vi "process.vi"(8 "error in (no error)":errorcluster, 9 "Calling VI Reference i":refnum<vi>, 10 "GObj Refnum":refnum<vi>, 11 "Loop in":refnum<class "Loop.lvclass">) -> (0 "error out":errorcluster, 3 "Loop out":refnum<class "Loop.lvclass">)   [LabVIEW 2016, in "Loop.lvclass"]
uses:
  Loop.lvclass
  C:/LSST_TS/SystemSW/ct_tools/GObject/GObject.lvclass
  Dependency/Dependency.lvclass
  DiagramObject/DiagramObject.lvclass
  GObject/GObject.lvclass/GObject.ctl
  DiagramObject/DiagramObject.lvclass/DiagramObject.ctl
  Dependency/Dependency.lvclass/Dependency.ctl
  GObject/GObject.lvclass
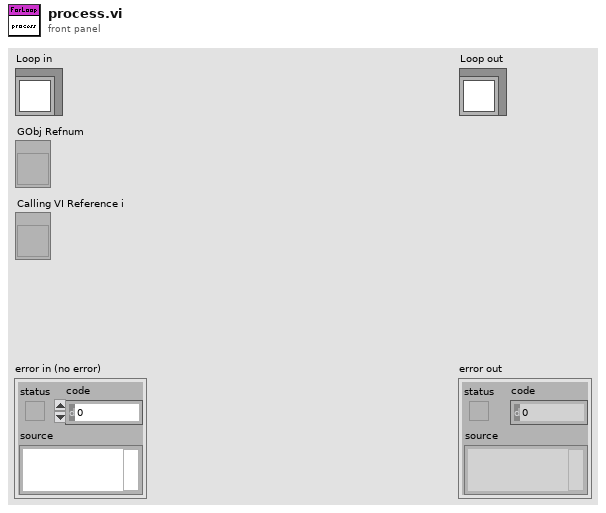
[diagram p1: front panel]
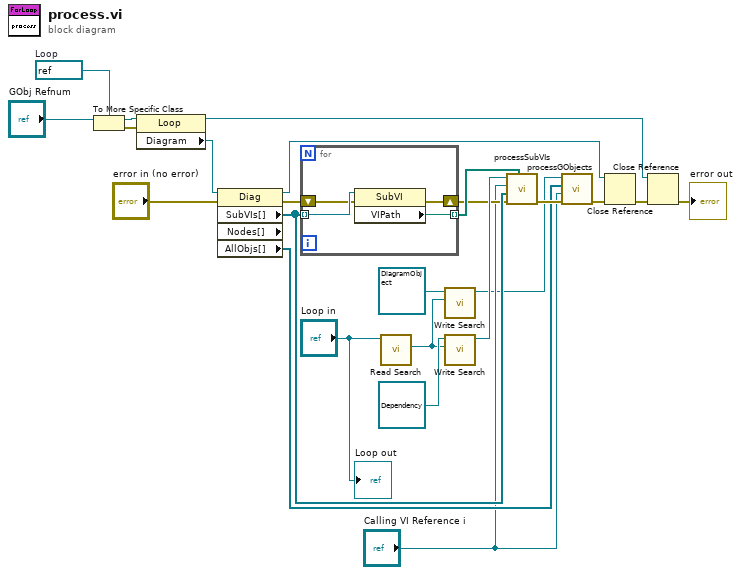
[diagram p0: block diagram]
diagram:
  w21 = refnum<vi> refnum  # Loop
  n1 = To More Specific Class(target class=w21, reference="GObj Refnum") -> (specific class reference=w24:refnum<vi>, error out=w23:errorcluster)  [unwired: 1 in]
  n2 = property class="Loop"(reference=w24, error in=w23) -> (reference out=w19:refnum<vi>, "Diagram"=w22:refnum<vi>)  [unwired: 1 out]
  n3 = property class="Diag" props=["SubVIs[]", "Nodes[]", "AllObjs[]"](reference=w22, error in="error in (no error)") -> (reference out=w13:refnum<vi>, error out=w10:errorcluster, "SubVIs[]"=w12:refnum<vi>[], "AllObjs[]"=w5:refnum<vi>[])  [unwired: 1 out]
  n4 = for {
    tunnel: w12 -> [w28] mode=indexing
    tunnel: [w27] -> w11 mode=indexing
    shift-right: [w26] -> w9
    shift-left: w10 -> [w25]
    n5 = property class="SubVI"(reference=w28, error in=w25) -> (error out=w26:errorcluster, "VIPath"=w27:path)  [unwired: 1 out]
  }
  n6 = call "Read Search.vi"("DiagramObject in"="Loop in") -> ("Search.lvclass"=w8:refnum<class "Search.lvclass">)  [unwired: 9 in, 1 out]
  n7 = call "Write Search.vi"("Search"=w8, "DiagramObject in"=refnum<class "DiagramObject.lvclass"> refnum ("DiagramObject.lvclass")) -> ("DiagramObject out"=w3:refnum<class "DiagramObject.lvclass">)  [unwired: 9 in]
  n8 = call "Write Search.vi"("Search"=w8, "Dependency in"=refnum<class "Dependency.lvclass"> refnum ("Dependency.lvclass")) -> ("Dependency out"=w17:refnum<class "Dependency.lvclass">)  [unwired: 9 in]
  n9 = call "processSubVIs.vi"("VIDependencyPaths"=w11, "error in (no error)"=w9, "SubVIs[]"=w12, "Calling VI Reference i"="Calling VI Reference i", "Dependency in"=w17) -> ("error out"=w6:errorcluster)  [unwired: 4 in, 2 out]
  n10 = call "processGObjects.vi"("error in (no error)"=w6, "Calling VI Reference i"="Calling VI Reference i", "All Objects[]"=w5, "DiagramObject in"=w3) -> ("error out"=w1:errorcluster)  [unwired: 6 in, 1 out]
  n11 = Close Reference(reference=w13, error in (no error)=w1) -> (error out=w20:errorcluster)
  n12 = Close Reference(reference=w19, error in (no error)=w20) -> (error out=→"error out":errorcluster)
  "Loop out" <- "Loop in"
